vi "Touched Lines.vi"(8 "error in (no error)":errorcluster, 11 "TermBuffer in":refnum<class "TermBuffer.lvclass">) -> (0 "error out":errorcluster, 2 "Touched Lines":bool[](array[boolean]), 3 "TermBuffer out":refnum<class "TermBuffer.lvclass">)   [LabVIEW 2020, in "Terminal.lvlib" / "TermBuffer.lvclass"]
uses:
  TermBuffer.lvclass
  TermBuffer.lvclass/TermBuffer.ctl
  TermLine/TermLine.lvclass
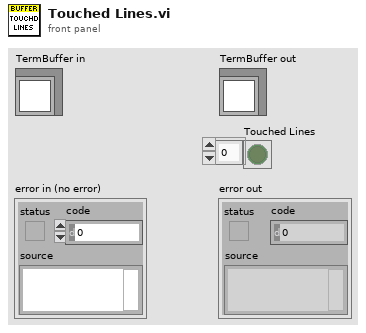
[diagram p1: front panel]
types:
  T1 = typedef "Terminal.lvlib/TermBuffer.lvclass/Ref Data.ctl" = cluster{"Lines":refnum<class "TermLine.lvclass">[], "Rows":i32, "Cols":i32}
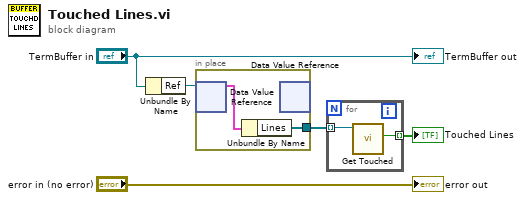
[diagram p0: block diagram]
diagram:
  n1 = Unbundle By Name("TermBuffer in") -> ("Ref"=w4:refnum<data-value>)
  n2 = in-place {
    in-place-border: [w6] -> w2
    n3 = in-place-dvr #1(w4) -> (w7:T1)  [unwired: 1 out]
    n4 = Unbundle By Name(w7) -> ("Lines"=w6:refnum<class "TermLine.lvclass">[])
    n5 = in-place-dvr #1() -> ()  [unwired: 1 in, 2 out]
  }
  n6 = for {
    tunnel: w2 -> [w9] mode=indexing
    tunnel: [w8] -> w1 mode=indexing
    n7 = call "Get Touched.vi"("TermLine in"=w9) -> ("Touched"=w8:bool)  [unwired: 8 in, 2 out]
  }
  "Touched Lines" <- w1
  "error out" <- "error in (no error)"
  "TermBuffer out" <- "TermBuffer in"
